vi "simple_run.vi"() -> ()   [LabVIEW 2016]
uses:
  Drivers/C8855-01/Transfer Mode.ctl
  Drivers/C8855-01/Trigger Mode.ctl
  <vilib>/DAQmx/write.llb/DAQmx Write (Analog Wfm 1Chan NSamp).vi
  <vilib>/DAQmx/create/channels.llb/DAQmx Create Channel (AO-Voltage-Basic).vi
  <vilib>/DAQmx/configure/timing.llb/DAQmx Timing (Sample Clock).vi
  <vilib>/DAQmx/miscellaneous.llb/DAQmx Fill In Error Info.vi
  <vilib>/DAQmx/create/channels.llb/DAQmx Create Channel (CO-Pulse Generation-Time).vi
  <vilib>/DAQmx/configure/timing.llb/DAQmx Timing (Implicit).vi
  <vilib>/DAQmx/configure/trigger.llb/DAQmx Start Trigger (Digital Edge).vi
  <vilib>/measure/NI_MABase.lvlib
  <resource>/objmgr/daqmx.rc
  Drivers/C8855-01/C8855-01.lvlib
panel:
  out "generated waveform":dbl[](array[numeric])
  out "pts to delay":i32
  out "cnt id":u8
  out "progress":dbl(slide) scale=0.0..1.0
  out "ampltiude":dbl
  out "# samples":i32
  out "sampling info":cluster{"Fs":dbl, "#s":dbl}
  out "trace":cluster{dbl[], "buffer out":u16[]}(graph)
  in  "offset":i32=5
  in  "range":i32=5
  in  "# repeats":i32=5
  in  "galvo freq (hz)":i32=10
  in  "gate time (us)":i32=500
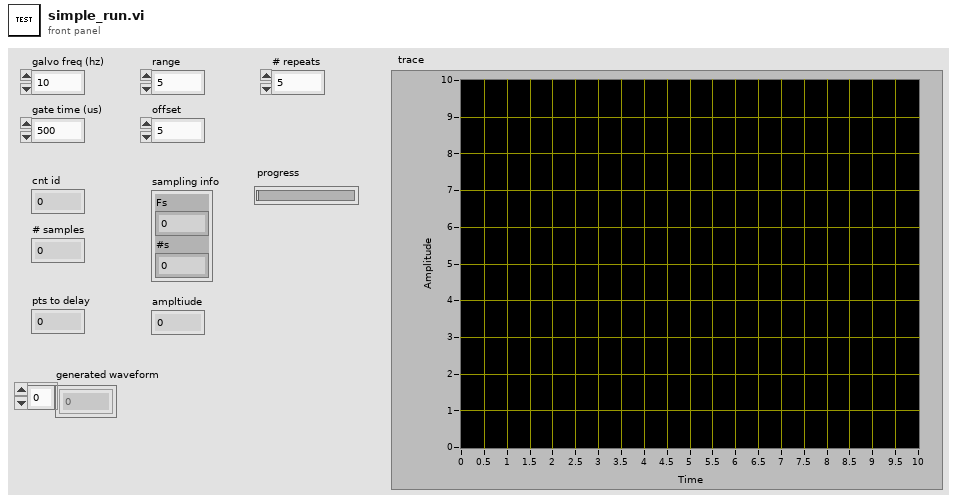
[diagram p1: front panel]
types:
  T1 = typedef "Drivers.lvlib/C8855-01.lvlib/Transfer Mode.ctl" = u8
  T2 = typedef "Drivers.lvlib/C8855-01.lvlib/Trigger Mode.ctl" = u8
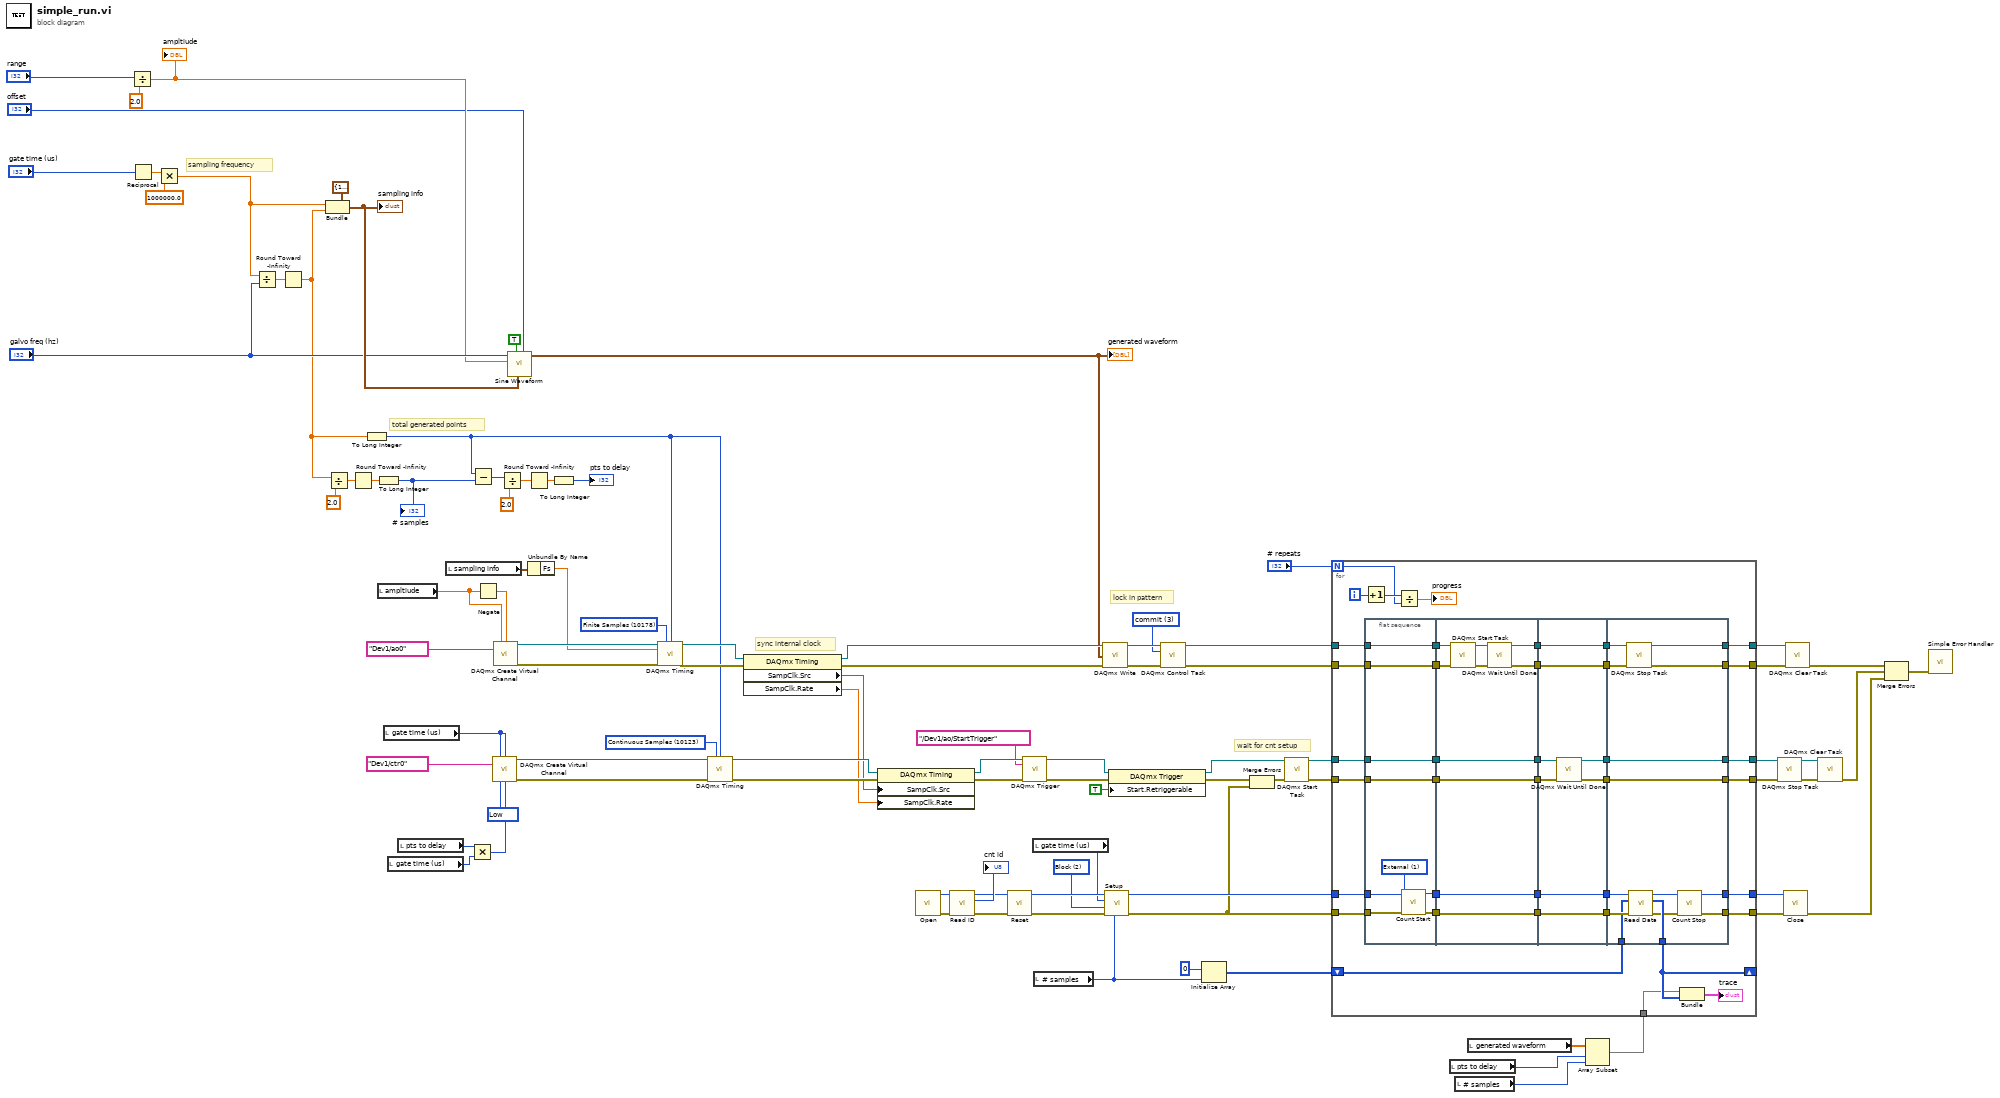
[diagram p0: block diagram]
diagram:
  w35 = T1 2 items=["Single"=1, "Block"=2] ("Transfer Mode")
  w50 = 3 items=["verify"=2, "reserve"=4, "commit"=3, "unreserve"=5, "abort"=6] ("action")
  w65 = 10214 items=["High"=10192, "Low"=10214] ("idle state")
  w66 = 10123 items=["Finite Samples"=10178, "Continuous Samples"=10123, "Hardware Timed Single Point"=12522] ("sample mode")
  w76 = 10178 items=["Finite Samples"=10178, "Continuous Samples"=10123, "Hardware Timed Single Point"=12522] ("sample mode")
  # "wait for cnt setup"
  # "lock in pattern"
  # "sync internal clock"
  # "total generated points"
  # "sampling frequency"
  n1 = Divide(x="range", y=2.0) -> (x/y=w89:dbl)
  "ampltiude" <- w89
  n2 = Reciprocal(x="gate time (us)") -> (1/x=w95:dbl)
  n3 = Multiply(x=w95, y=1000000.0) -> (x*y=w88:dbl)
  n4 = Divide(x=w88, y="galvo freq (hz)") -> (x/y=w87:dbl)
  n5 = Round Toward -Infinity(1:w87) -> (0:w75:dbl)
  n6 = Bundle(cluster=cluster{"Fs":dbl, "#s":dbl} {"Fs"=1000.0, "#s"=1000.0} ("sampling info"), "Fs"=w88, "#s"=w75) -> (w97:cluster{"Fs":dbl, "#s":dbl})
  "sampling info" <- w97
  n7 = Divide(x=w75, y=2.0) -> (x/y=w84:dbl)
  n8 = Round Toward -Infinity(1:w84) -> (0:w82:dbl)
  n9 = To Long Integer(number=w75) -> (32bit integer=w15:i32)
  n10 = To Long Integer(number=w82) -> (32bit integer=w14:i32)
  "# samples" <- w14
  n11 = local read "ampltiude"() -> (w80:dbl)
  n12 = local read "gate time (us)"() -> (w67:i32)
  n13 = local read "gate time (us)"() -> (w3:i32)
  n14 = local read "pts to delay"() -> (w2:i32)
  n15 = local read "sampling info"() -> (w74:cluster{"Fs":dbl, "#s":dbl})
  n16 = Multiply(x=w2, y=w3) -> (x*y=w1:i32)
  n17 = Subtract(x=w15, y=w14) -> (x-y=w13:i32)
  n18 = Negate(x=w80) -> (-x=w79:dbl)
  n19 = call-poly <vilib>:"DAQmx Create Virtual Channel.vi"("high time"=w67, "low time"=w67, "counter"=tag "Dev1/ctr0", "idle state"=w65, "initial delay"=w1) -> ("task out"=w70:refnum<k21>, "error out"=w69:errorcluster)  [unwired: 9 in]
  n20 = call-poly <vilib>:"DAQmx Create Virtual Channel.vi"("maximum value"=w80, "minimum value"=w79, "physical channels"=tag "Dev1/ao0") -> ("task out"=w78:refnum<k21>, "error out"=w77:errorcluster)  [unwired: 11 in]
  n21 = Divide(x=w13, y=2.0) -> (x/y=w11:dbl)
  n22 = call <vilib>:"Sine Waveform.vi"("offset"="offset", "sampling info"=w97, "reset signal"=TRUE, "amplitude"=w89, "frequency"="galvo freq (hz)") -> ("signal out"=w8:waveform(dbl))  [unwired: 5 in, 1 out]
  "generated waveform" <- w8
  n23 = Round Toward -Infinity(1:w11) -> (0:w10:dbl)
  n24 = Unbundle By Name(w74) -> ("Fs"=w73:dbl)
  n25 = To Long Integer(number=w10) -> (32bit integer=→"pts to delay":i32)
  n26 = call-poly <vilib>:"DAQmx Timing.vi"("task/channels in"=w78, "sample mode"=w76, "samples per channel"=w15, "rate"=w73, "error in"=w77) -> ("task out"=w71:refnum<k21>, "error out"=w72:errorcluster)  [unwired: 9 in]
  n27 = call-poly <vilib>:"DAQmx Timing.vi"("task/channels in"=w70, "sample mode"=w66, "samples per channel"=w15, "error in"=w69) -> ("task out"=w63:refnum<k21>, "error out"=w64:errorcluster)  [unwired: 10 in]
  n28 = property class="DAQmx Timing"(reference=w71, error in=w72) -> (reference out=w53:refnum<k21>, error out=w54:errorcluster, "SampClk.Src"=w62:tag, "SampClk.Rate"=w61:dbl)
  n29 = property class="DAQmx Timing"(reference=w63, error in=w64, "SampClk.Src"=w62, "SampClk.Rate"=w61) -> (reference out=w59:refnum<k21>, error out=w60:errorcluster)
  n30 = call "Open.vi"() -> ("error out"=w42:errorcluster, "Handle"=w43:u32)  [unwired: 10 in]
  n31 = call "Read ID.vi"("error in (no error)"=w42, "handle in"=w43) -> ("error out"=w38:errorcluster, "ID"=→"cnt id":u8, "handle out"=w39:u32)  [unwired: 7 in]
  n32 = call "Reset.vi"("error in (no error)"=w38, "handle in"=w39) -> ("error out"=w36:errorcluster, "handle out"=w37:u32)  [unwired: 8 in]
  n33 = call-poly <vilib>:"DAQmx Trigger.vi"("task/channels in"=w59, "source"=tag "/Dev1/ao/StartTrigger", "error in"=w60) -> ("task out"=w56:refnum<k21>, "error out"=w57:errorcluster)  [unwired: 11 in]
  n34 = local read "gate time (us)"() -> (w34:i32)
  n35 = local read "# samples"() -> (w31:i32)
  n36 = call-poly <vilib>:"DAQmx Write.vi"("task/channels in"=w53, "data"=w8, "error in"=w54) -> ("task out"=w51:refnum<k21>, "error out"=w52:errorcluster)  [unwired: 10 in, 1 out]
  n37 = call "Setup.vi"("Number of Gate"=w31, "error in (no error)"=w36, "Transfer Mode"=w35, "Gate Time (us)"=w34, "Handle"=w37) -> ("error out"=w28:errorcluster, "Handle out"=w29:u32)  [unwired: 5 in]
  n38 = property class="DAQmx Trigger"(reference=w56, error in=w57, "Start.Retriggerable"=TRUE) -> (reference out=w48:refnum<k21>, error out=w49:errorcluster)
  n39 = call <vilib>:"DAQmx Control Task.vi"("task/channels in"=w51, "action"=w50, "error in"=w52) -> ("task out"=w44:refnum<k21>, "error out"=w45:errorcluster)  [unwired: 11 in]
  n40 = Initialize Array(u16 0 ("element"), w31) -> (w30:u16[])
  n41 = Merge Errors(w49, w28) -> (w33:errorcluster)
  n42 = call <vilib>:"DAQmx Start Task.vi"("task/channels in"=w48, "error in"=w33) -> ("task out"=w46:refnum<k21>, "error out"=w47:errorcluster)  [unwired: 12 in]
  n43 = local read "pts to delay"() -> (w6:i32)
  n44 = local read "# samples"() -> (w5:i32)
  n45 = local read "generated waveform"() -> (w7:dbl[])
  n46 = Array Subset(array=w7, index=w6, length=w5) -> (w4:dbl[])
  n47 = for {
    N: "# repeats" -> [w123]
    tunnel: w46 -> [w131]
    tunnel: w44 -> [w134]
    tunnel: w29 -> [w119]
    tunnel: [w111] -> w27
    shift-right: [w100] -> _
    shift-left: w30 -> [w110]
    tunnel: w28 -> [w116]
    tunnel: [w115] -> w26
    tunnel: w47 -> [w129]
    tunnel: [w113] -> w25
    tunnel: w45 -> [w135]
    tunnel: [w114] -> w20
    tunnel: [w102] -> w24
    tunnel: [w101] -> w21
    tunnel: w4 -> [w98]
    i -> [w125]
    n48 = Increment(x=w125) -> (x+1=w124:i32)
    n49 = flat-sequence {
      tunnel: w116 -> [w137]
      tunnel: w119 -> [w138]
      tunnel: w129 -> [w141]
      tunnel: w131 -> [w142]
      tunnel: w134 -> [w143]
      tunnel: w135 -> [w144]
      tunnel: [w144] -> w109
      tunnel: [w143] -> w108
      tunnel: [w142] -> w107
      tunnel: [w141] -> w106
      tunnel: [w139] -> w105
      tunnel: [w140] -> w104
      tunnel: [w150] -> w133
      tunnel: [w149] -> w132
      tunnel: [w148] -> w130
      tunnel: [w147] -> w128
      tunnel: [w146] -> w120
      tunnel: [w145] -> w117
      tunnel: w109 -> [w154]
      tunnel: w108 -> [w153]
      tunnel: w107 -> [w148]
      tunnel: w106 -> [w147]
      tunnel: w105 -> [w146]
      tunnel: w104 -> [w145]
      tunnel: w133 -> [w162]
      tunnel: w132 -> [w161]
      tunnel: w130 -> [w160]
      tunnel: w128 -> [w159]
      tunnel: [w162] -> w127
      tunnel: [w161] -> w126
      tunnel: [w158] -> w121
      tunnel: w120 -> [w158]
      tunnel: [w157] -> w118
      tunnel: w117 -> [w157]
      tunnel: [w156] -> w112
      tunnel: [w155] -> w103
      tunnel: w127 -> [w175]
      tunnel: w126 -> [w176]
      tunnel: w121 -> [w174]
      tunnel: w118 -> [w173]
      tunnel: [w166] -> w115
      tunnel: [w172] -> w114
      tunnel: [w171] -> w113
      tunnel: w112 -> [w171]
      tunnel: [w167] -> w111
      tunnel: w110 -> [w170]
      tunnel: [w169] -> w100
      tunnel: w103 -> [w164]
      tunnel: [w164] -> w102
      tunnel: [w163] -> w101
      frame #0 {
        w136 = T2 1 items=["Software", "External"] ("Trigger Mode")
        n50 = call "Count Start.vi"("error in (no error)"=w137, "Trigger Mode"=w136, "handle in"=w138) -> ("error out"=w140:errorcluster, "handle out"=w139:u32)  [unwired: 7 in]
      }
      frame #1 {
        n51 = call <vilib>:"DAQmx Start Task.vi"("task/channels in"=w153, "error in"=w154) -> ("task out"=w152:refnum<k21>, "error out"=w151:errorcluster)  [unwired: 12 in]
        n52 = call <vilib>:"DAQmx Wait Until Done.vi"("task/channels in"=w152, "error in"=w151) -> ("task out"=w149:refnum<k21>, "error out"=w150:errorcluster)  [unwired: 12 in]
      }
      frame #2 {
        n53 = call <vilib>:"DAQmx Wait Until Done.vi"("task/channels in"=w160, "error in"=w159) -> ("task out"=w155:refnum<k21>, "error out"=w156:errorcluster)  [unwired: 12 in]
      }
      frame #3 {
        n54 = call <vilib>:"DAQmx Stop Task.vi"("task/channels in"=w176, "error in"=w175) -> ("task out"=w163:refnum<k21>, "error out"=w172:errorcluster)  [unwired: 12 in]
        n55 = call "Read Data.vi"("error in (no error)"=w173, "buffer in"=w170, "handle in"=w174) -> ("error out"=w165:errorcluster, "buffer out"=w169:u16[], "handle out"=w168:u32)  [unwired: 6 in]
        n56 = call "Count Stop.vi"("error in (no error)"=w165, "handle in"=w168) -> ("error out"=w166:errorcluster, "handle out"=w167:u32)  [unwired: 8 in]
      }
    }
    n57 = Divide(x=w124, y=w123) -> (x/y=→"progress":dbl)
    n58 = Bundle(w98, "buffer out"=w100) -> (→"trace":cluster{dbl[], "buffer out":u16[]})  [unwired: 1 in]
  }
  n59 = call <vilib>:"DAQmx Stop Task.vi"("task/channels in"=w24, "error in"=w25) -> ("task out"=w22:refnum<k21>, "error out"=w23:errorcluster)  [unwired: 12 in]
  n60 = call "Close.vi"("error in (no error)"=w26, "handle in"=w27) -> ("error out"=w17:errorcluster)  [unwired: 9 in]
  n61 = call <vilib>:"DAQmx Clear Task.vi"("task in"=w21, "error in"=w20) -> ("error out"=w19:errorcluster)  [unwired: 13 in]
  n62 = call <vilib>:"DAQmx Clear Task.vi"("task in"=w22, "error in"=w23) -> ("error out"=w18:errorcluster)  [unwired: 13 in]
  n63 = Merge Errors(w19, w18, w17) -> (w16:errorcluster)
  n64 = call <vilib>:"Simple Error Handler.vi"("error in (no error)"=w16) -> ()  [unwired: 4 in, 5 out]
